vi "IT7800 ACQ.vi"(8 "error in":errorcluster, 10 "Read selection":T3, 11 "VISA in":refnum<visa-resource-name>="TCPIP::192.168.0.252::INSTR") -> (0 "error out":errorcluster, 1 "PSU Values 3PH":T1, 2 "PSU Values":T2, 3 "VISA out":refnum<visa-resource-name>, 5 "3 PHase":bool)   [LabVIEW 2025]
uses:
  TypeDefs/Psu1PhaseValues.ctl
  TypeDefs/Psu3PhaseValues.ctl
  <vilib>/Instr/_visa.llb/VISA Flush IO Buffer Mask.ctl
  <instrlib>/IT7800/IT7800.lvlib
panel:
  out "Run counter":u32
  out "Response Energy":string
  out "Response Power":string
  out "Response [ms]":dbl format="%.2g"
  out "Response Basic":string
  # "In 3phase system values are \naverage of all three phases"
  # "IP7800 Driver V0.13\nAcquisition"
  # "21.05.2025"
  # "Andrej Valand"
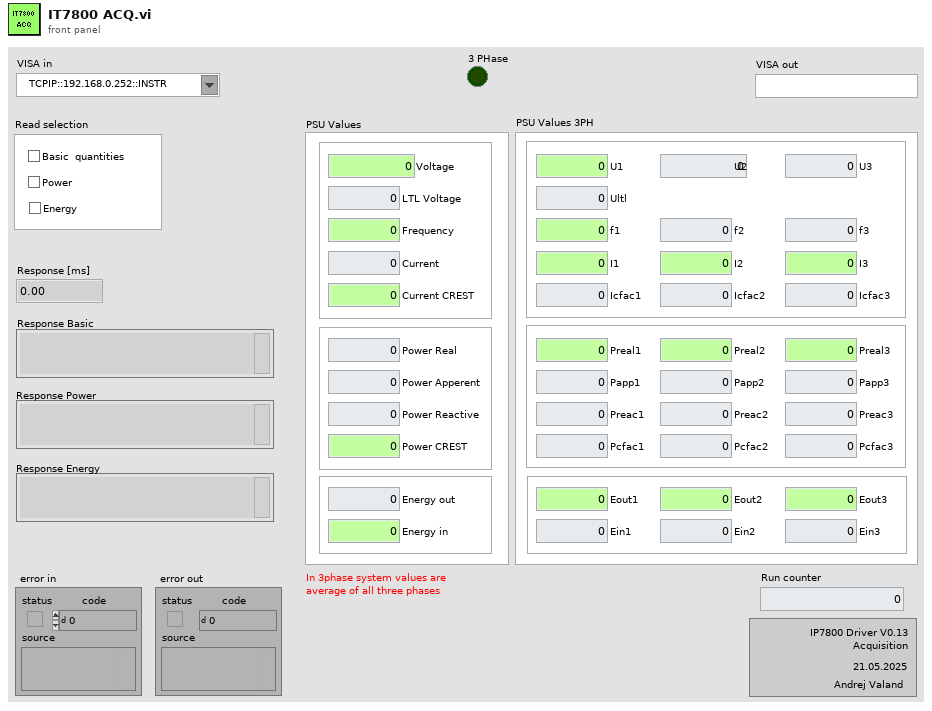
[diagram p1: front panel]
types:
  T1 = typedef "Psu3PhaseValues.ctl" = cluster{"U1":dbl, "U2":dbl, "U3":dbl, "Ultl":dbl, "f1":dbl, "f2":dbl, "f3":dbl, "I1":dbl, "I2":dbl, "I3":dbl, "Icfac1":dbl, "Icfac2":dbl, "Icfac3":dbl, "Preal1":dbl, "Preal2":dbl, "Preal3":dbl, "Papp1":dbl, "Papp2":dbl, "Papp3":dbl, "Preac1":dbl, "Preac2":dbl, "Preac3":dbl, "Pcfac1":dbl, "Pcfac2":dbl, "Pcfac3":dbl, "Eout1":dbl, "Eout2":dbl, "Eout3":dbl, "Ein1":dbl, "Ein2":dbl, "Ein3":dbl}
  T2 = typedef "Psu1PhaseValues.ctl" = cluster{"Voltage":dbl, "LTL Voltage":dbl, "Frequency":dbl, "Current":dbl, "Current CREST":dbl, "Power Real":dbl, "Power Apperent":dbl, "Power Reactive":dbl, "Power CREST":dbl, "Energy out":dbl, "Energy in":dbl}
  T3 = cluster{"Basic  quantities":bool, "Power":bool, "Energy":bool}
  T4 = typedef "VISA Flush IO Buffer Mask.ctl" = u16
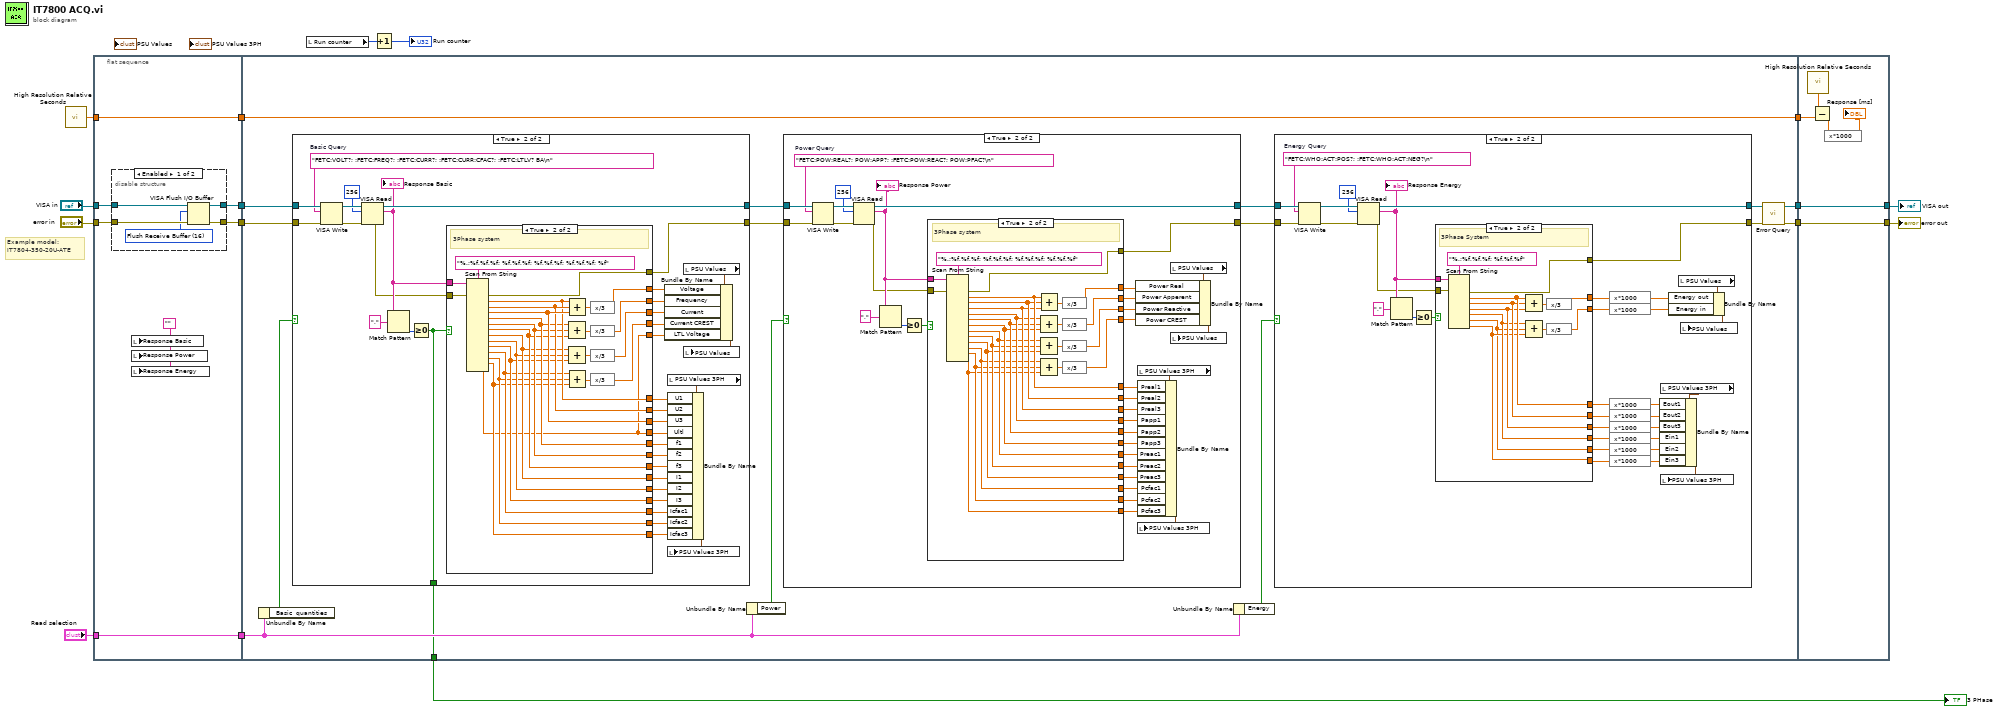
[diagram p0: block diagram]
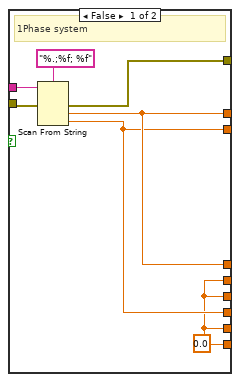
[diagram p4: hidden frame]
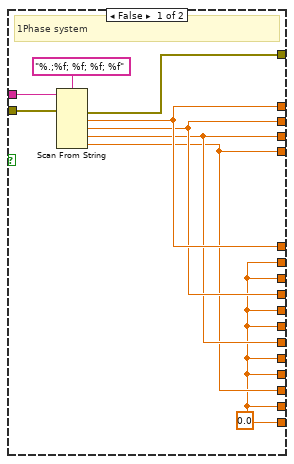
[diagram p6: hidden frame]
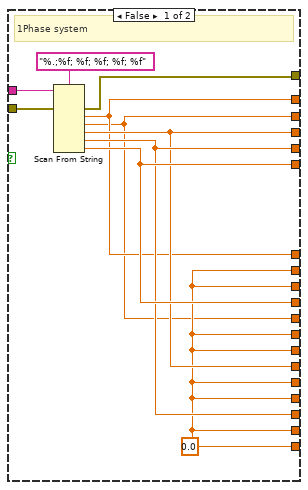
[diagram p8: hidden frame]
diagram:
  # "Example model:\nIT7804-350-20U-ATE"
  n1 = call <vilib>:"High Resolution Relative Seconds.vi"() -> ("relative seconds"=w2:dbl)
  n2 = flat-sequence {
    tunnel: "error in" -> [w19]
    tunnel: "VISA in" -> [w20]
    tunnel: [w18] -> w14
    tunnel: [w17] -> w13
    tunnel: [w21] -> w12
    tunnel: [w23] -> w10
    tunnel: "Read selection" -> [w23]
    tunnel: w2 -> [w21]
    tunnel: w14 -> [w46]
    tunnel: w13 -> [w45]
    tunnel: w12 -> [w44]
    tunnel: [w44] -> w11
    tunnel: w10 -> [w38]
    tunnel: [w33] -> w8
    tunnel: [w32] -> w7
    tunnel: [w31] -> w1
    tunnel: w11 -> [w247]
    tunnel: [w246] -> w6
    tunnel: w8 -> [w246]
    tunnel: [w245] -> w5
    tunnel: w7 -> [w245]
    frame #0 {
      w22 = ""
      n3 = disable-structure shown="Enabled" {
        disable-tunnel: w20 -> [w28 w30]
        disable-tunnel: w19 -> [w27 w29]
        disable-tunnel: [w26 w30] -> w18
        disable-tunnel: [w25 w29] -> w17
        frame Enabled {
          w24 = T4 16 items=["Flush Receive Buffer"=16, "Write Transmit Buffer to Device"=32, "Flush Receive Buffer (No I/O)"=64, "Flush Transmit Buffer"=128] ("Mask")
          n4 = VISA Flush I/O Buffer(VISA resource name=w28, mask (16)=w24, error in (no error)=w27) -> (VISA resource name out=w26:refnum<visa-resource-name>, error out=w25:errorcluster)
        }
        frame Disabled {
        }
      }
      n5 = local write "Response Basic"(w22) -> ()
      n6 = local write "Response Power"(w22) -> ()
      n7 = local write "Response Energy"(w22) -> ()
    }
    frame #1 {
      n8 = Unbundle By Name(w38) -> ("Basic  quantities"=w43:bool)
      n9 = case shown="True" w43 {
        tunnel: w46 -> [w172 w204]
        tunnel: w45 -> [w171 w203]
        tunnel: [w172 w201] -> w41
        tunnel: [w171 w178] -> w40
        tunnel: [_ w173] -> w31
        frame False {
        }
        frame True {
          w202 = "FETC:VOLT?; :FETC:FREQ?; :FETC:CURR?; :FETC:CURR:CFAC?; :FETC:LTLV? BA\n"  # Basic Query
          n10 = VISA Write(VISA resource name=w204, write buffer=w202, error in (no error)=w203) -> (VISA resource name out=w207:refnum<visa-resource-name>, error out=w206:errorcluster)  [unwired: 1 out]
          n11 = VISA Read(VISA resource name=w207, byte count=u32 256, error in (no error)=w206) -> (VISA resource name out=w201:refnum<visa-resource-name>, read buffer=w180:string, error out=w179:errorcluster)  [unwired: 1 out]
          "Response Basic" <- w180
          n12 = Match Pattern(string=w180, regular expression=",") -> (offset past match=w187:i32)  [unwired: 1 in, 3 out]
          n13 = Greater Or Equal To 0?(x=w187) -> (x >= 0?=w173:bool)
          n14 = case shown="True" w173 {
            tunnel: [w211 w232] -> w182
            tunnel: [w210 w231] -> w183
            tunnel: [w213 w226] -> w184
            tunnel: [w214 w224] -> w185
            tunnel: [w215 w220] -> w186
            tunnel: w180 -> [w216 w242]
            tunnel: [w211 w238] -> w188
            tunnel: [w212 w239] -> w189
            tunnel: [w212 w240] -> w190
            tunnel: [w215 w220] -> w191
            tunnel: [w210 w235] -> w192
            tunnel: [w212 w234] -> w193
            tunnel: [w212 w233] -> w194
            tunnel: [w213 w229] -> w195
            tunnel: [w212 w228] -> w196
            tunnel: [w212 w227] -> w197
            tunnel: [w214 w223] -> w198
            tunnel: [w212 w222] -> w199
            tunnel: [w212 w221] -> w200
            tunnel: w179 -> [w209 w219]
            tunnel: [w208 w218] -> w178
            frame False {
              w212 = 0.0
              # "1Phase system"
              n15 = Scan From String(format string="%.;%f; %f; %f; %f; %f", input string=w216, error in=w209) -> (error out=w208:errorcluster, output 1=w211:dbl, output 2=w210:dbl, output 3=w213:dbl, output 4=w214:dbl, output 5=w215:dbl)  [unwired: 6 in, 2 out]
            }
            frame True {
              # "3Phase system"
              n16 = Scan From String(format string="%.;%f,%f,%f; %f,%f,%f; %f,%f,%f; %f,%f,%f; %f", input string=w242, error in=w219) -> (error out=w218:errorcluster, output 1=w238:dbl, output 2=w239:dbl, output 3=w240:dbl, output 4=w235:dbl, output 5=w234:dbl, output 6=w233:dbl, output 7=w229:dbl, output 8=w228:dbl, output 9=w227:dbl, output 10=w223:dbl, output 11=w222:dbl, output 12=w221:dbl, output 13=w220:dbl)  [unwired: 14 in, 2 out]
              n17 = Compound Arithmetic op=ADD(w235, w234, w233) -> (w236:dbl)
              n18 = Compound Arithmetic op=ADD(w229, w228, w227) -> (w230:dbl)
              n19 = Compound Arithmetic op=ADD(w238, w239, w240) -> (w237:dbl)
              n20 = Compound Arithmetic op=ADD(w223, w222, w221) -> (w225:dbl)
              n21 = expression code="x/3"(w236) -> (w231:dbl)
              n22 = expression code="x/3"(w230) -> (w226:dbl)
              n23 = expression code="x/3"(w237) -> (w232:dbl)
              n24 = expression code="x/3"(w225) -> (w224:dbl)
            }
          }
          n25 = local read "PSU Values 3PH"() -> (w175:T1)
          n26 = Bundle By Name(cluster=w175, "U1"=w188, "U2"=w189, "U3"=w190, "Ultl"=w191, "f1"=w192, "f2"=w193, "f3"=w194, "I1"=w195, "I2"=w196, "I3"=w197, "Icfac1"=w198, "Icfac2"=w199, "Icfac3"=w200) -> (w174:T1)
          n27 = local write "PSU Values 3PH"(w174) -> ()
          n28 = local read "PSU Values"() -> (w177:T2)
          n29 = Bundle By Name(cluster=w177, "Voltage"=w182, "Frequency"=w183, "Current"=w184, "Current CREST"=w185, "LTL Voltage"=w186) -> (w176:T2)
          n30 = local write "PSU Values"(w176) -> ()
        }
      }
      n31 = Unbundle By Name(w38) -> ("Power"=w42:bool)
      n32 = case shown="True" w42 {
        tunnel: w41 -> [w104 w134]
        tunnel: w40 -> [w103 w133]
        tunnel: [w104 w131] -> w37
        tunnel: [w103 w109] -> w36
        frame False {
        }
        frame True {
          w132 = "FETC:POW:REAL?; POW:APP?; :FETC:POW:REAC?; POW:PFAC?\n"  # Power Query
          n33 = VISA Write(VISA resource name=w134, write buffer=w132, error in (no error)=w133) -> (VISA resource name out=w137:refnum<visa-resource-name>, error out=w136:errorcluster)  [unwired: 1 out]
          n34 = VISA Read(VISA resource name=w137, byte count=u32 256, error in (no error)=w136) -> (VISA resource name out=w131:refnum<visa-resource-name>, read buffer=w111:string, error out=w110:errorcluster)  [unwired: 1 out]
          "Response Power" <- w111
          n35 = Match Pattern(string=w111, regular expression=",") -> (offset past match=w113:i32)  [unwired: 1 in, 3 out]
          n36 = Greater Or Equal To 0?(x=w113) -> (x >= 0?=w114:bool)
          n37 = case shown="True" w114 {
            tunnel: [w144 w152] -> w115
            tunnel: [w143 w151] -> w116
            tunnel: [w142 w150] -> w117
            tunnel: [w141 w149] -> w118
            tunnel: w111 -> [w145 w170]
            tunnel: [w144 w167] -> w119
            tunnel: [w143 w163] -> w120
            tunnel: [w142 w160] -> w121
            tunnel: [w141 w155] -> w122
            tunnel: [w140 w153] -> w123
            tunnel: [w140 w154] -> w124
            tunnel: [w140 w158] -> w125
            tunnel: [w140 w159] -> w126
            tunnel: [w140 w161] -> w127
            tunnel: [w140 w162] -> w128
            tunnel: [w140 w165] -> w129
            tunnel: [w140 w166] -> w130
            tunnel: w110 -> [w139 w148]
            tunnel: [w138 w147] -> w109
            frame False {
              w140 = 0.0
              # "1Phase system"
              n38 = Scan From String(format string="%.;%f; %f; %f; %f", input string=w145, error in=w139) -> (error out=w138:errorcluster, output 1=w144:dbl, output 2=w143:dbl, output 3=w142:dbl, output 4=w141:dbl)  [unwired: 5 in, 2 out]
            }
            frame True {
              # "3Phase system"
              n39 = Scan From String(format string="%.;%f,%f,%f; %f,%f,%f; %f,%f,%f; %f,%f,%f", input string=w170, error in=w148) -> (error out=w147:errorcluster, output 1=w167:dbl, output 2=w166:dbl, output 3=w165:dbl, output 4=w163:dbl, output 5=w162:dbl, output 6=w161:dbl, output 7=w160:dbl, output 8=w159:dbl, output 9=w158:dbl, output 10=w155:dbl, output 11=w154:dbl, output 12=w153:dbl)  [unwired: 13 in, 2 out]
              n40 = Compound Arithmetic op=ADD(w163, w162, w161) -> (w164:dbl)
              n41 = Compound Arithmetic op=ADD(w160, w159, w158) -> (w156:dbl)
              n42 = Compound Arithmetic op=ADD(w155, w154, w153) -> (w157:dbl)
              n43 = Compound Arithmetic op=ADD(w167, w166, w165) -> (w168:dbl)
              n44 = expression code="x/3"(w164) -> (w151:dbl)
              n45 = expression code="x/3"(w156) -> (w150:dbl)
              n46 = expression code="x/3"(w157) -> (w149:dbl)
              n47 = expression code="x/3"(w168) -> (w152:dbl)
            }
          }
          n48 = local read "PSU Values 3PH"() -> (w106:T1)
          n49 = Bundle By Name(cluster=w106, "Preal1"=w119, "Preal2"=w130, "Preal3"=w129, "Papp1"=w120, "Papp2"=w128, "Papp3"=w127, "Preac1"=w121, "Preac2"=w126, "Preac3"=w125, "Pcfac1"=w122, "Pcfac2"=w124, "Pcfac3"=w123) -> (w105:T1)
          n50 = local write "PSU Values 3PH"(w105) -> ()
          n51 = local read "PSU Values"() -> (w108:T2)
          n52 = Bundle By Name(cluster=w108, "Power Real"=w115, "Power Apperent"=w116, "Power Reactive"=w117, "Power CREST"=w118) -> (w107:T2)
          n53 = local write "PSU Values"(w107) -> ()
        }
      }
      n54 = Unbundle By Name(w38) -> ("Energy"=w39:bool)
      n55 = case shown="True" w39 {
        tunnel: w37 -> [w48 w78]
        tunnel: w36 -> [w47 w77]
        tunnel: [w48 w75] -> w35
        tunnel: [w47 w59] -> w34
        frame False {
        }
        frame True {
          w76 = "FETC:WHO:ACT:POS?; :FETC:WHO:ACT:NEG?\n"  # Energy Query
          n56 = VISA Write(VISA resource name=w78, write buffer=w76, error in (no error)=w77) -> (VISA resource name out=w81:refnum<visa-resource-name>, error out=w80:errorcluster)  [unwired: 1 out]
          n57 = VISA Read(VISA resource name=w81, byte count=u32 256, error in (no error)=w80) -> (VISA resource name out=w75:refnum<visa-resource-name>, read buffer=w61:string, error out=w60:errorcluster)  [unwired: 1 out]
          "Response Energy" <- w61
          n58 = Match Pattern(string=w61, regular expression=",") -> (offset past match=w65:i32)  [unwired: 1 in, 3 out]
          n59 = Greater Or Equal To 0?(x=w65) -> (x >= 0?=w66:bool)
          n60 = case shown="True" w66 {
            tunnel: w61 -> [w87 w102]
            tunnel: [w86 w92] -> w67
            tunnel: [w85 w91] -> w68
            tunnel: [w86 w98] -> w69
            tunnel: [w85 w95] -> w70
            tunnel: [w84 w94] -> w71
            tunnel: [w84 w93] -> w72
            tunnel: [w84 w96] -> w73
            tunnel: [w84 w97] -> w74
            tunnel: w60 -> [w83 w90]
            tunnel: [w82 w89] -> w59
            frame False {
              w84 = 0.0
              # "1Phase system"
              n61 = Scan From String(format string="%.;%f; %f", input string=w87, error in=w83) -> (error out=w82:errorcluster, output 1=w86:dbl, output 2=w85:dbl)  [unwired: 3 in, 2 out]
            }
            frame True {
              # "3Phase System"
              n62 = Scan From String(format string="%.;%f,%f,%f; %f,%f,%f", input string=w102, error in=w90) -> (error out=w89:errorcluster, output 1=w98:dbl, output 2=w97:dbl, output 3=w96:dbl, output 4=w95:dbl, output 5=w93:dbl, output 6=w94:dbl)  [unwired: 7 in, 2 out]
              n63 = Compound Arithmetic op=ADD(w98, w97, w96) -> (w100:dbl)
              n64 = Compound Arithmetic op=ADD(w95, w93, w94) -> (w99:dbl)
              n65 = expression code="x/3"(w100) -> (w92:dbl)
              n66 = expression code="x/3"(w99) -> (w91:dbl)
            }
          }
          n67 = expression code="x*1000"(w67) -> (w56:dbl)
          n68 = expression code="x*1000"(w68) -> (w55:dbl)
          n69 = expression code="x*1000"(w69) -> (w54:dbl)
          n70 = expression code="x*1000"(w74) -> (w49:dbl)
          n71 = expression code="x*1000"(w73) -> (w50:dbl)
          n72 = expression code="x*1000"(w70) -> (w53:dbl)
          n73 = expression code="x*1000"(w72) -> (w51:dbl)
          n74 = expression code="x*1000"(w71) -> (w52:dbl)
          n75 = local read "PSU Values 3PH"() -> (w58:T1)
          n76 = Bundle By Name(cluster=w58, "Eout1"=w54, "Eout2"=w49, "Eout3"=w50, "Ein1"=w53, "Ein2"=w51, "Ein3"=w52) -> (w57:T1)
          n77 = local write "PSU Values 3PH"(w57) -> ()
          n78 = local read "PSU Values"() -> (w63:T2)
          n79 = Bundle By Name(cluster=w63, "Energy out"=w56, "Energy in"=w55) -> (w62:T2)
          n80 = local write "PSU Values"(w62) -> ()
        }
      }
      n81 = call <instrlib>:"Error Query.vi"("error in"=w34, "VISA resource name"=w35) -> ("error out"=w32:errorcluster, "VISA resource name out"=w33:refnum<visa-resource-name>)  [unwired: 6 in, 2 out]
    }
    frame #2 {
      n82 = call <vilib>:"High Resolution Relative Seconds.vi"() -> ("relative seconds"=w248:dbl)
      n83 = Subtract(x=w248, y=w247) -> (x-y=w244:dbl)
      n84 = expression code="x*1000"(w244) -> (→"Response [ms]":dbl)
    }
  }
  n85 = local read "Run counter"() -> (w4:u32)
  n86 = Increment(x=w4) -> (x+1=→"Run counter":u32)
  "error out" <- w5
  "VISA out" <- w6
  "3 PHase" <- w1
